vi "access table insert sqlite.vi"(6 "SQLite Password":string, 8 "error in (no error)":errorcluster, 9 "Access Password":string, 10 "table":string, 11 "路径":path) -> (0 "错误输出":errorcluster, 3 "条数":i32)   [LabVIEW 2016]
uses:
  <vilib>/addons/database/Connection.llb/DB Tools Open Connec (String).vi
  <vilib>/addons/database/NI_Database_API.lvlib
  SQLite/SQLite Lib.lvlib
  Access/Access Lib.lvlib
panel:
  out "名称":string
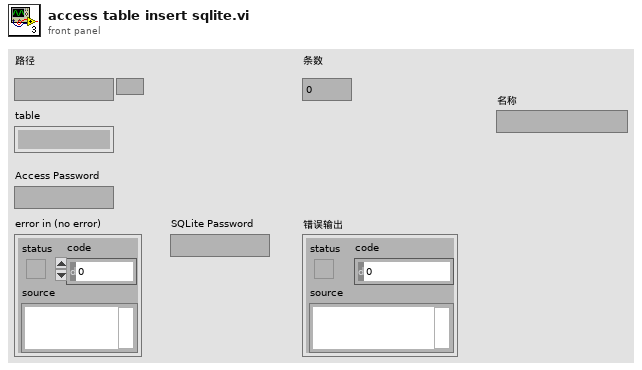
[diagram p1: front panel]
types:
  T1 = cluster{"columns外部输入":bool, "columns input":string[]}
  T2 = typedef "NI_Database_API.lvlib/Conn ObjectReference.ctl" = refnum<k1>
  T3 = typedef "NI_Database_API.lvlib/DB Tools DataTypes.ctl" = enum16{"String", "Long (I32)", "Single (SGL)", "Double (DBL)", "Date/Time", "Binary"}
  T4 = cluster{"name":string, "database data type":T3, "defined size":i32}[]
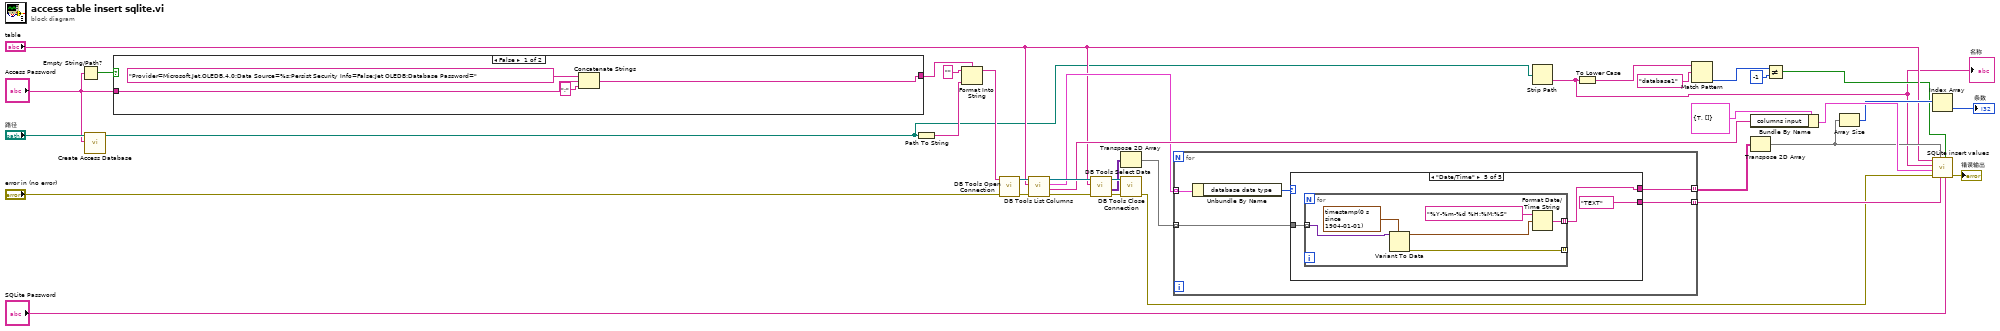
[diagram p0: block diagram]
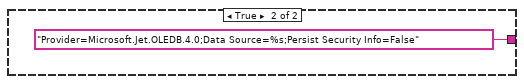
[diagram p2: hidden frame]
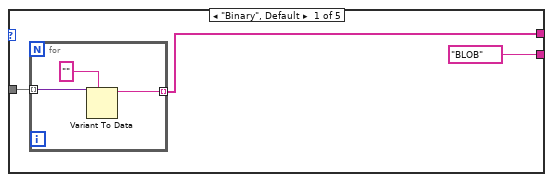
[diagram p3: hidden frame]
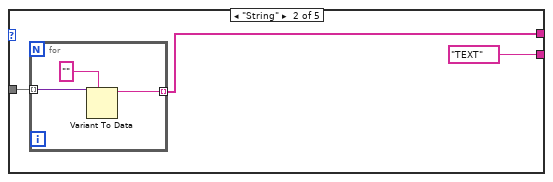
[diagram p4: hidden frame]
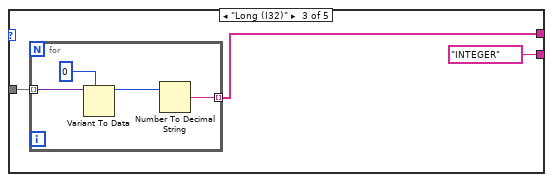
[diagram p5: hidden frame]
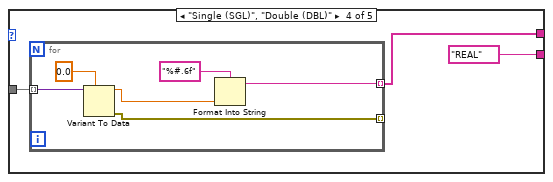
[diagram p6: hidden frame]
diagram:
  n1 = Empty String/Path?(string/path="Access Password") -> (empty?=w9:bool)
  n2 = call "Create Access Database.vi"("Password"="Access Password", "路径"="路径") -> ("路径 out"=w3:path)  [unwired: 8 in, 1 out]
  n3 = case shown="False" w9 {
    tunnel: [w37 "Provider=Microsoft.Jet.OLEDB.4.0;Data Source=%s;Persist Security Info=False" ("格式字符串")] -> w8
    tunnel: "Access Password" -> [w40 _]
    frame False {
      n4 = Concatenate Strings("Provider=Microsoft.Jet.OLEDB.4.0;Data Source=%s;Persist Security Info=False;Jet OLEDB:Database Password=" ("格式字符串"), w40, ";" ("字符串")) -> (w37:string)
    }
    frame True {
    }
  }
  n5 = Path To String(path=w3) -> (string=w6:string)
  n6 = Format Into String(format string=w8, initial string="" ("初始字符串"), w6) -> (resulting string=w4:string)  [unwired: 1 in, 1 out]
  n7 = call-poly <vilib>:"DB Tools Open Connection.vi"("error in (no error)"="error in (no error)", "connection information"=w4) -> ("error out"=w32:errorcluster, "connection reference"=w36:T2)  [unwired: 6 in]
  n8 = call <vilib>:"DB Tools List Columns.vi"("error in (no error)"=w32, "table"="table", "connection reference"=w36) -> ("error out"=w31:errorcluster, "columns"=w28:string[], "column information"=w27:T4, "connection reference out"=w33:T2)  [unwired: 1 in]
  n9 = call <vilib>:"DB Tools Select Data.vi"("error in (no error)"=w31, "table"="table", "connection reference"=w33) -> ("error out"=w34:errorcluster, "data"=w25:variant[][], "connection reference out"=w35:T2)  [unwired: 3 in]
  n10 = Transpose 2D Array(2D array=w25) -> (transposed array=w24:variant[][])
  n11 = call <vilib>:"DB Tools Close Connection.vi"("error in (no error)"=w34, "connection reference"=w35) -> ("error out"=w22:errorcluster)  [unwired: 5 in]
  n12 = for {
    tunnel: w27 -> [w46] mode=indexing
    tunnel: [w44] -> w26 mode=indexing
    tunnel: w24 -> [w43] mode=indexing
    tunnel: [w42] -> w23 mode=indexing
    n13 = Unbundle By Name(w46) -> ("database data type"=w45:T3)
    n14 = case shown="\"Date/Time\"" w45 {
      tunnel: ["BLOB" ("组合框") "TEXT" ("组合框") "INTEGER" ("组合框") "REAL" ("组合框") "TEXT" ("组合框")] -> w44
      tunnel: w43 -> [w48 w54 w60 w67 w76]
      tunnel: [w47 w53 w59 w66 w75] -> w42
      frame "Binary", Default {
        n15 = for {
          tunnel: w48 -> [w51] mode=indexing
          tunnel: [w50] -> w47 mode=indexing
          n16 = Variant To Data(type="", Variant=w51) -> (data=w50:string)  [unwired: 1 in, 1 out]
        }
      }
      frame "String" {
        n17 = for {
          tunnel: w54 -> [w57] mode=indexing
          tunnel: [w56] -> w53 mode=indexing
          n18 = Variant To Data(type="", Variant=w57) -> (data=w56:string)  [unwired: 1 in, 1 out]
        }
      }
      frame "Long (I32)" {
        n19 = for {
          tunnel: w60 -> [w63] mode=indexing
          tunnel: [w62] -> w59 mode=indexing
          n20 = Variant To Data(type=0, Variant=w63) -> (data=w65:i32)  [unwired: 1 in, 1 out]
          n21 = Number To Decimal String(number=w65) -> (decimal integer string=w62:string)  [unwired: 1 in]
        }
      }
      frame "Single (SGL)", "Double (DBL)" {
        n22 = for {
          tunnel: w67 -> [w71] mode=indexing
          tunnel: [w70] -> w66 mode=indexing
          tunnel: [w69] -> _ mode=indexing
          n23 = Variant To Data(type=sgl 0.0, Variant=w71) -> (data=w73:sgl, error out=w69:errorcluster)  [unwired: 1 in]
          n24 = Format Into String(format string="%#.6f" ("格式字符串"), w73) -> (resulting string=w70:string)  [unwired: 2 in, 1 out]
        }
      }
      frame "Date/Time" {
        n25 = for {
          tunnel: w76 -> [w81] mode=indexing
          tunnel: [w79] -> w75 mode=indexing
          tunnel: [w78] -> _ mode=indexing
          n26 = Variant To Data(type=timestamp(0 s since 1904-01-01) ("时间标识"), Variant=w81) -> (data=w80:timestamp, error out=w78:errorcluster)  [unwired: 1 in]
          n27 = Format Date/Time String(time format string (%c)="%Y-%m-%d %H:%M:%S" ("时间格式字符串(%c)"), seconds (now)=w80) -> (date/time string=w79:string)  [unwired: 1 in]
        }
      }
    }
  }
  n28 = Strip Path(path=w3) -> (name=w11:string)  [unwired: 1 out]
  "名称" <- w11
  n29 = To Lower Case(string=w11) -> (all lower case string=w10:string)
  n30 = Match Pattern(string=w10, regular expression="database1" ("正则表达式")) -> (offset past match=w14:i32)  [unwired: 1 in, 3 out]
  n31 = Bundle By Name(cluster=T1 {"columns外部输入"=TRUE, "columns input"=[]} ("columns外部输入"), "columns input"=w28) -> (w29:T1)
  n32 = Transpose 2D Array(2D array=w23) -> (transposed array=w19:string[][])
  n33 = Not Equal?(x=w14, y=-1) -> (x != y?=w12:bool)
  n34 = Array Size(array=w19) -> (size(s)=w18:i32[])
  n35 = Index Array(array=w18) -> (element=→"条数":i32)  [unwired: 1 in]
  n36 = call "SQLite insert values.vi"("Password"="SQLite Password", "是否创建唯一键"=w12, "columns  INFO"=w26, "数组"=w19, "错误输入（无错误）"=w22, "columns外部输入"=w29, "database"=w11, "Tabe Name"="table") -> ("错误输出"=→"错误输出":errorcluster)  [unwired: 3 in]
